vi "Populate Entry Details.vi"(8 "error in":errorcluster, 9 "Sub-Index":string, 10 "Index":string, 11 "Object Dictionary UI in":refnum<class "Object Dictionary UI.lvclass">) -> (0 "error out":errorcluster, 3 "Object Dictionary UI out":refnum<class "Object Dictionary UI.lvclass">)   [LabVIEW 2024, in "Object Dictionary UI.lvlib" / "Object Dictionary UI.lvclass"]
uses:
  Object Dictionary UI.lvclass
  Object Dictionary UI.lvclass/Object Dictionary UI.ctl
  EDS-File-Viewer/Core/Access SRDO.ctl
  EDS-File-Viewer/Core/Electronic Datasheet.lvlib
  EDS-File-Viewer/Core/Access PDO.ctl
  EDS-File-Viewer/Core/Access SDO.ctl
  EDS-File-Viewer/Core/Object Type.ctl
  EDS-File-Viewer/Electronic Datasheet/Electronic Datasheet.lvclass
  EDS-File-Viewer/Core/OD Entry/OD Entry.lvclass
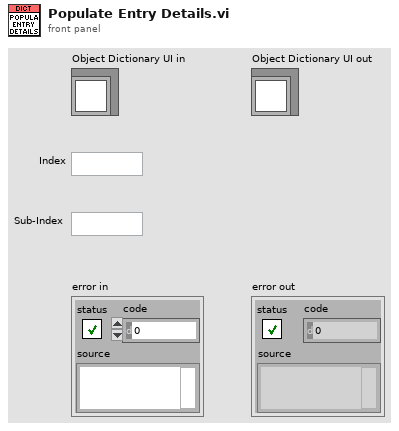
[diagram p1: front panel]
types:
  T1 = typedef "Electronic Datasheet.lvlib/Access SDO.ctl" = enum16{"read only", "write only", "read/write", "read/write on process input", "read/write on process output", "constant value", "UNKNOWN"}
  T2 = typedef "Electronic Datasheet.lvlib/Object Type.ctl" = u8
  T3 = typedef "Electronic Datasheet.lvlib/Access PDO.ctl" = enum16{"no", "t", "r", "tr"}
  T4 = typedef "Electronic Datasheet.lvlib/Access SRDO.ctl" = enum16{"no", "tx", "rx", "trx"}
  T5 = cluster{"Index":string, "Sub-Index":string, "ParameterName":string, "Denotation":string, "Description":string, "ObjectType":T2, "HighLimit":string, "DataType":u16, "LowLimit":string, "Access SDO":T1, "Access PDO":T3, "Access SRDO":T4, "DefaultValue":string}
  T6 = enum16{"ro", "wo", "rw", "rwr", "rww", "const", "UNKNOWN"}
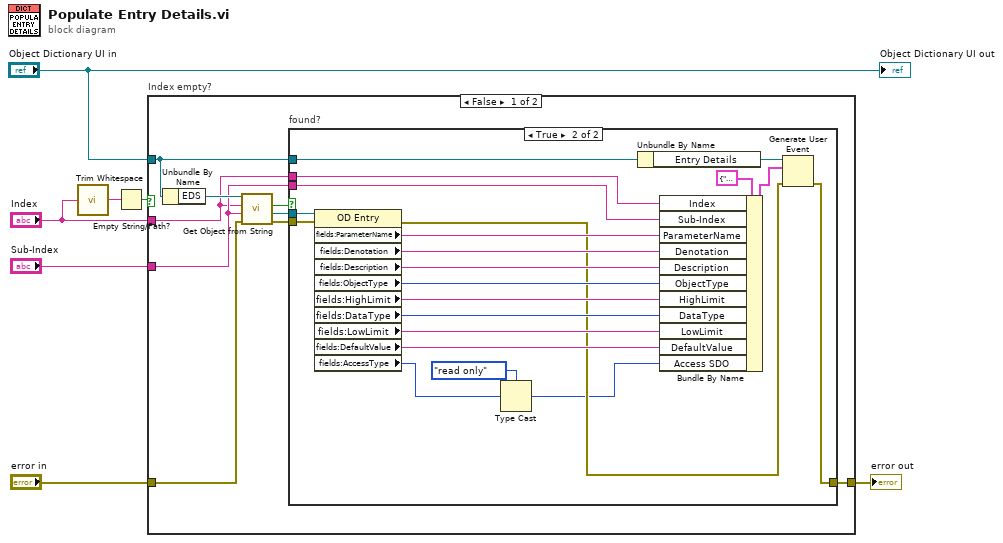
[diagram p0: block diagram]
diagram:
  n1 = call <vilib>:"Trim Whitespace.vi"("string"="Index") -> ("trimmed string"=w2:string)  [unwired: 1 in]
  n2 = Empty String/Path?(string/path=w2) -> (empty?=w3:bool)
  n3 = case "Index empty?" shown="False" w3 {
    tunnel: [w16 w39] -> w7
    tunnel: "Object Dictionary UI in" -> [w15 _]
    tunnel: "error in" -> [w13 w39]
    tunnel: "Sub-Index" -> [w10 _]
    tunnel: "Index" -> [w9 _]
    frame False {
      n4 = Unbundle By Name(w15) -> ("EDS"=w14:refnum<class "Electronic Datasheet.lvclass">)
      n5 = call "Get Object from String.vi"("error in"=w13, "Sub-Index"=w10, "Index"=w9, "reference in"=w14) -> ("error out"=w8:errorcluster, "OD Entry"=w11:refnum<class "OD Entry.lvclass">, "Found?"=w12:bool)  [unwired: 4 in, 1 out]
      n6 = case "found?" shown="True" w12 {
        tunnel: [w17 w35] -> w16
        tunnel: w15 -> [_ w34]
        tunnel: w11 -> [_ w33]
        tunnel: w10 -> [_ w32]
        tunnel: w9 -> [_ w31]
        tunnel: w8 -> [w17 w22]
        frame False {
        }
        frame True {
          n7 = property class="OD Entry"(reference=w33, error in=w22) -> (error out=w21:errorcluster, "fields:ParameterName"=w30:string, "fields:Denotation"=w29:string, "fields:Description"=w28:string, "fields:ObjectType"=w27:T2, "fields:HighLimit"=w26:string, "fields:DataType"=w25:u16, "fields:LowLimit"=w24:string, "fields:DefaultValue"=w23:string, "fields:AccessType"=w18:T6)  [unwired: 1 out]
          n8 = Type Cast(type=Access_SDO."read only" ("Access SDO"), x=w18) -> (*(type *) &x=w19:T1)
          n9 = Unbundle By Name(w34) -> ("Entry Details"=w38:refnum<user-event>)
          n10 = Bundle By Name(cluster=T5 {"Index"="", "Sub-Index"="", "ParameterName"="", "Denotation"="", "Description"="", "ObjectType"=0, "HighLimit"="", "DataType"=0, "LowLimit"="", "Access SDO"=enum."read only", "Access PDO"=enum."no", "Access SRDO"=enum."no", "DefaultValue"=""} ("event data"), "Index"=w31, "Sub-Index"=w32, "ParameterName"=w30, "Denotation"=w29, "Description"=w28, "ObjectType"=w27, "HighLimit"=w26, "DataType"=w25, "LowLimit"=w24, "DefaultValue"=w23, "Access SDO"=w19) -> (w36:T5)
          n11 = Generate User Event(user event=w38, event data cluster=w36, error in=w21) -> (error out=w35:errorcluster)  [unwired: 1 in, 1 out]
        }
      }
    }
    frame True {
    }
  }
  "error out" <- w7
  "Object Dictionary UI out" <- "Object Dictionary UI in"
